vi "Set Target Field.vi"(1 "error in":T2, 2 "Target Field (kG)":dbl format="%.3f", 3 "Communications Config":T1={"GPIB address"=22, "GPIB bus"=0, "connection ID"=refnum, "IP"="192.168.2.200", "Active Comm Interface"=0, "Serial Port"="", "Programmer Type"=0} {"Programmer Type" items=["Model 430", "Model 420"]; "Active Comm Interface" items=["TCP/IP (Model 430 Only)", "RS232", "IEEE488"]}) -> (0 "error out":T2)   [LabVIEW 2018]
panel:
  in  "GPIB Address":cluster{"GPIB address":i16, "GPIB bus":i16}={"GPIB address"=22, "GPIB bus"=0}
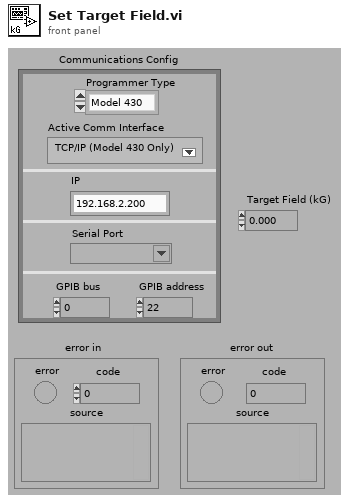
[diagram p1: front panel]
types:
  T1 = cluster{"GPIB address":i16, "GPIB bus":i16, "connection ID":refnum<k5>, "IP":string, "Active Comm Interface":u16, "Serial Port":refnum<visa-resource-name>, "Programmer Type":u16}
  T2 = cluster{"error":bool, "code":i32, "source":string}
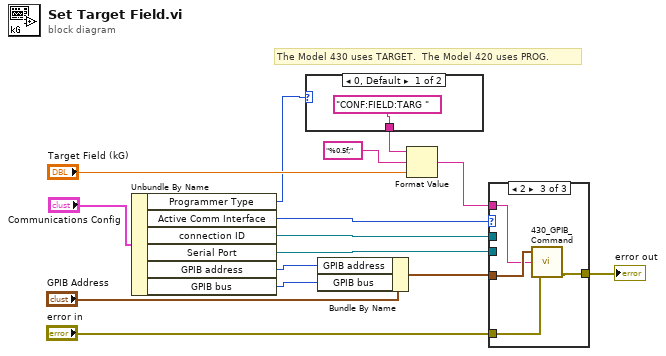
[diagram p0: block diagram]
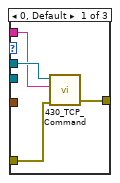
[diagram p2: hidden frame]
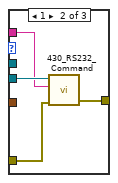
[diagram p3: hidden frame]
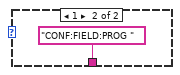
[diagram p4: hidden frame]
diagram:
  # "The Model 430 uses TARGET.  The Model 420 uses PROG."
  n1 = Unbundle By Name("Communications Config") -> ("Programmer Type"=w1:u16, "Active Comm Interface"=w3:u16, "connection ID"=w9:refnum<k5>, "Serial Port"=w8:refnum<visa-resource-name>, "GPIB address"=w11:i16, "GPIB bus"=w12:i16)
  n2 = case shown="0, Default" w1 {
    tunnel: ["CONF:FIELD:TARG " "CONF:FIELD:PROG "] -> w15
    frame 0, Default {
    }
    frame 1 {
    }
  }
  n3 = Bundle By Name(cluster="GPIB Address", "GPIB address"=w11, "GPIB bus"=w12) -> (w7:cluster{"GPIB address":i16, "GPIB bus":i16})
  n4 = Format Value(string ("")=w15, format string="%0.5f;", value (0)="Target Field (kG)") -> (output string=w5:string)
  n5 = case shown="2" w3 {
    tunnel: [w21 w25 w29] -> w4
    tunnel: w7 -> [_ _ w28]
    tunnel: w9 -> [w20 _ _]
    tunnel: w8 -> [_ w24 _]
    tunnel: w5 -> [w19 w23 w27]
    tunnel: "error in" -> [w18 w22 w26]
    frame 0, Default {
      n6 = call "430_TCP_Command.vi"("error in (no error)"=w18, "Command"=w19, "connection ID"=w20) -> ("error out"=w21:errorcluster)  [unwired: 1 in, 2 out]
    }
    frame 1 {
      n7 = call "430_RS232_Command.vi"("error in (no error)"=w22, "Command"=w23, "VISA resource name"=w24) -> ("error out"=w25:errorcluster)  [unwired: 1 in, 2 out]
    }
    frame 2 {
      n8 = call "430_GPIB_Command.vi"("GPIB (In)"=w28, "Input command"=w27, "error in"=w26) -> ("error out"=w29:T2)  [unwired: 3 out]
    }
  }
  "error out" <- w4
